vi "例8.2 有限模入.vi"() -> ()   [LabVIEW 2017]
uses:
  <vilib>/DAQmx/read.llb/DAQmx Read (Analog 2D DBL NChan NSamp).vi
  <vilib>/DAQmx/create/channels.llb/DAQmx Create Channel (AI-Voltage-Basic).vi
  <vilib>/DAQmx/configure/timing.llb/DAQmx Timing (Sample Clock).vi
  <vilib>/DAQmx/miscellaneous.llb/DAQmx Fill In Error Info.vi
panel:
  out "波形图":dbl[][](graph)
  in  "number of samples per channel":i32=1000 caption="每通道采样数"
  in  "samples per channel":i32=1000 caption="每通道采样"
  in  "sample mode":i32(ring)=10178 caption="采样模式" items=["有限采样"=10178, "连续采样"=10123, "硬件定时单点"=12522]
  in  "rate":dbl=1000.0 caption="采样率" format="%0.2f"
  in  "name to assign":string caption="分配名称"
  in  "input terminal configuration":i32(ring)=-1 caption="输入接线端配置" items=["默认"=-1, "RSE"=10083, "NRSE"=10078, "差分"=10106, "伪差分"=12529]
  in  "maximum value":dbl=5.0 caption="最大值" format="%0.2f"
  in  "minimum value":dbl=-5.0 caption="最小值" format="%0.2f"
  in  "physical channels":tag caption="物理通道"
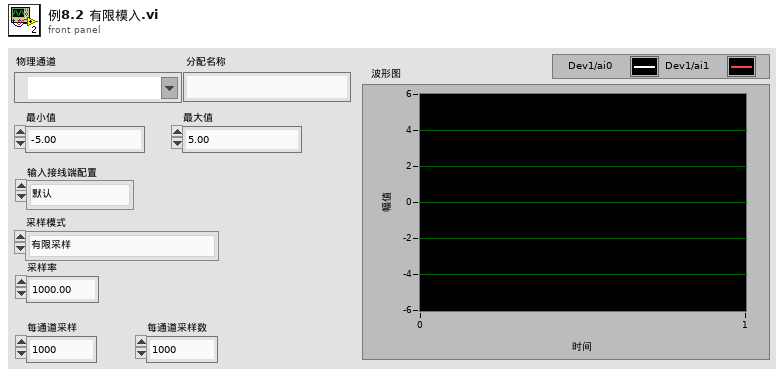
[diagram p1: front panel]
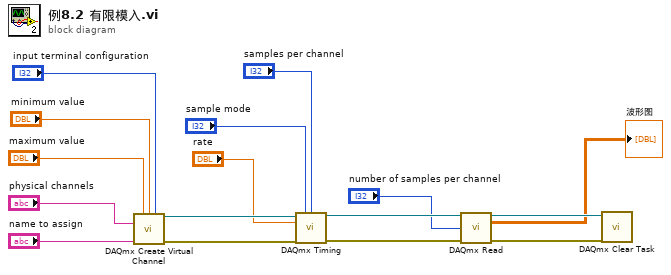
[diagram p0: block diagram]
diagram:
  n1 = call-poly <vilib>:"DAQmx Create Virtual Channel.vi"("maximum value"="maximum value", "minimum value"="minimum value", "input terminal configuration"="input terminal configuration", "physical channels"="physical channels", "name to assign"="name to assign") -> ("task out"=w16:refnum<k21>, "error out"=w13:errorcluster)  [unwired: 9 in]
  n2 = call-poly <vilib>:"DAQmx Timing.vi"("task/channels in"=w16, "sample mode"="sample mode", "samples per channel"="samples per channel", "rate"="rate", "error in"=w13) -> ("task out"=w15:refnum<k21>, "error out"=w12:errorcluster)  [unwired: 9 in]
  n3 = call-poly <vilib>:"DAQmx Read.vi"("task/channels in"=w15, "number of samples per channel"="number of samples per channel", "error in"=w12) -> ("task out"=w14:refnum<k21>, "data"=→"波形图":dbl[][], "error out"=w11:errorcluster)  [unwired: 10 in]
  n4 = call <vilib>:"DAQmx Clear Task.vi"("task in"=w14, "error in"=w11) -> ()  [unwired: 13 in, 1 out]
